vi "Version information to VIP API Version.vi"(8 "error in (no error)":errorcluster, 10 "Bitness String":string, 11 "Version String":string) -> (0 "error out":errorcluster, 3 "VIP Version":string)   [LabVIEW 2011, in "G CLI VIP.lvlib"]
uses:
  G CLI VIP.lvlib
  <vilib>/regexp/Match Regular Expression.xnode
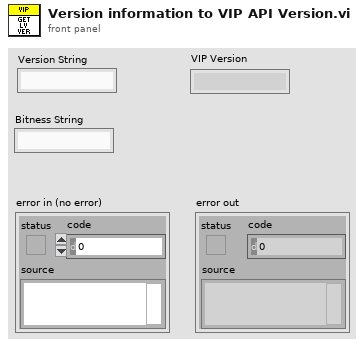
[diagram p1: front panel]
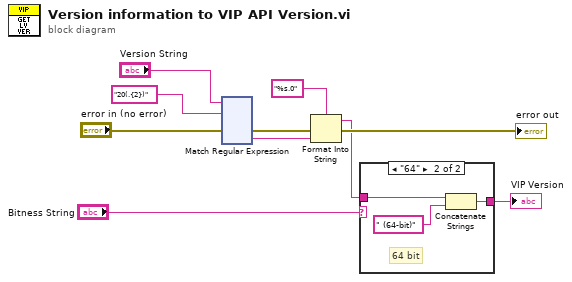
[diagram p0: block diagram]
diagram:
  n1 = xnode "Match Regular Expression"("input string"="Version String", "regular expression"="20(.{2})", "error in"="error in (no error)") -> ("error out"=w7:errorcluster, "submatch 1"=w6:string)  [unwired: 3 in, 4 out]
  n2 = Format Into String(format string="%s.0", error in=w7, w6) -> (resulting string=w3:string, error out=→"error out":errorcluster)  [unwired: 1 in]
  n3 = case shown="\"64\"" "Bitness String" {
    tunnel: w3 -> [w11 w14]
    tunnel: [w11 w13] -> w2
    frame Default {
      # "32 bit"
    }
    frame "64" {
      # "64 bit"
      n4 = Concatenate Strings(w14, " (64-bit)" ("string")) -> (w13:string)
    }
  }
  "VIP Version" <- w2
